vi "Custom Failure Message.vi"() -> ()   [LabVIEW 2017, in "Assertion.Tests.lvlib" / "Assert Not Refnum.lvlib"]
uses:
  Assert Not Refnum.lvlib
  Assertion/Assertion.lvlib
panel:
  out "error out":errorcluster
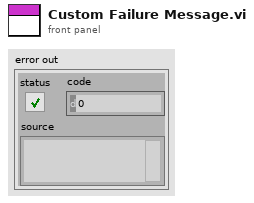
[diagram p1: front panel]
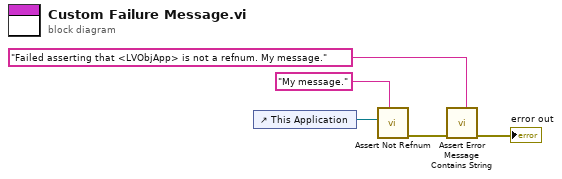
[diagram p0: block diagram]
diagram:
  n1 = control-ref of="This Application"() -> (w3:refnum<vi>)
  n2 = call "Assert Not Refnum.vi"("Message (\"\")"="My message." ("Message (\"\")"), "Refnum"=w3) -> ("error out"=w5:errorcluster)  [unwired: 9 in]
  n3 = call "Assert Error Message Contains String.vi"("Expected"="Failed asserting that <LVObjApp> is not a refnum. My message.", "error in (no error)"=w5) -> ("error out"=→"error out":errorcluster)  [unwired: 9 in]
